vi "AddConstantPower.vi"(0 "deviceName":string, 1 "channel":u8, 2 "repeats":u16=1, 3 "power":sgl, 4 "samplingInterval":sgl, 5 "maxDuration":sgl, 6 "maxVoltage":sgl=inf, 7 "error in (no error)":errorcluster, 8 "isMaximumVoltageVsOCP":bool, 9 "minVoltage":sgl=-inf, 10 "isMinimumVoltageVsOCP":bool, 11 "maxCurrent":sgl=inf, 12 "minCurrent":sgl=-inf, 13 "maxCapacity":sgl=inf) -> (27 "error out":errorcluster)   [LabVIEW 2018]
doc: "EXPORT void AisAddConstantPower(const char* deviceName, uint8_t channel, uint16_t repeats, float power, float samplingInterval, float maxDuration, float maxVoltage, bool isMaximumVoltageVsOCP, float minVoltage, bool isMinimumVoltageVsOCP, float maxCurrent, float minCurrent, float maxCapacity);"
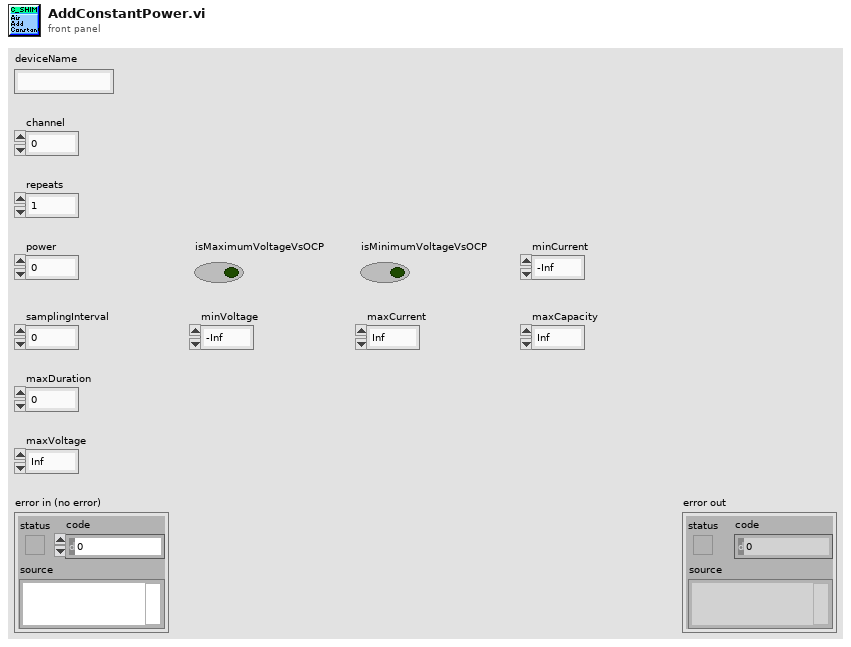
[diagram p1: front panel]
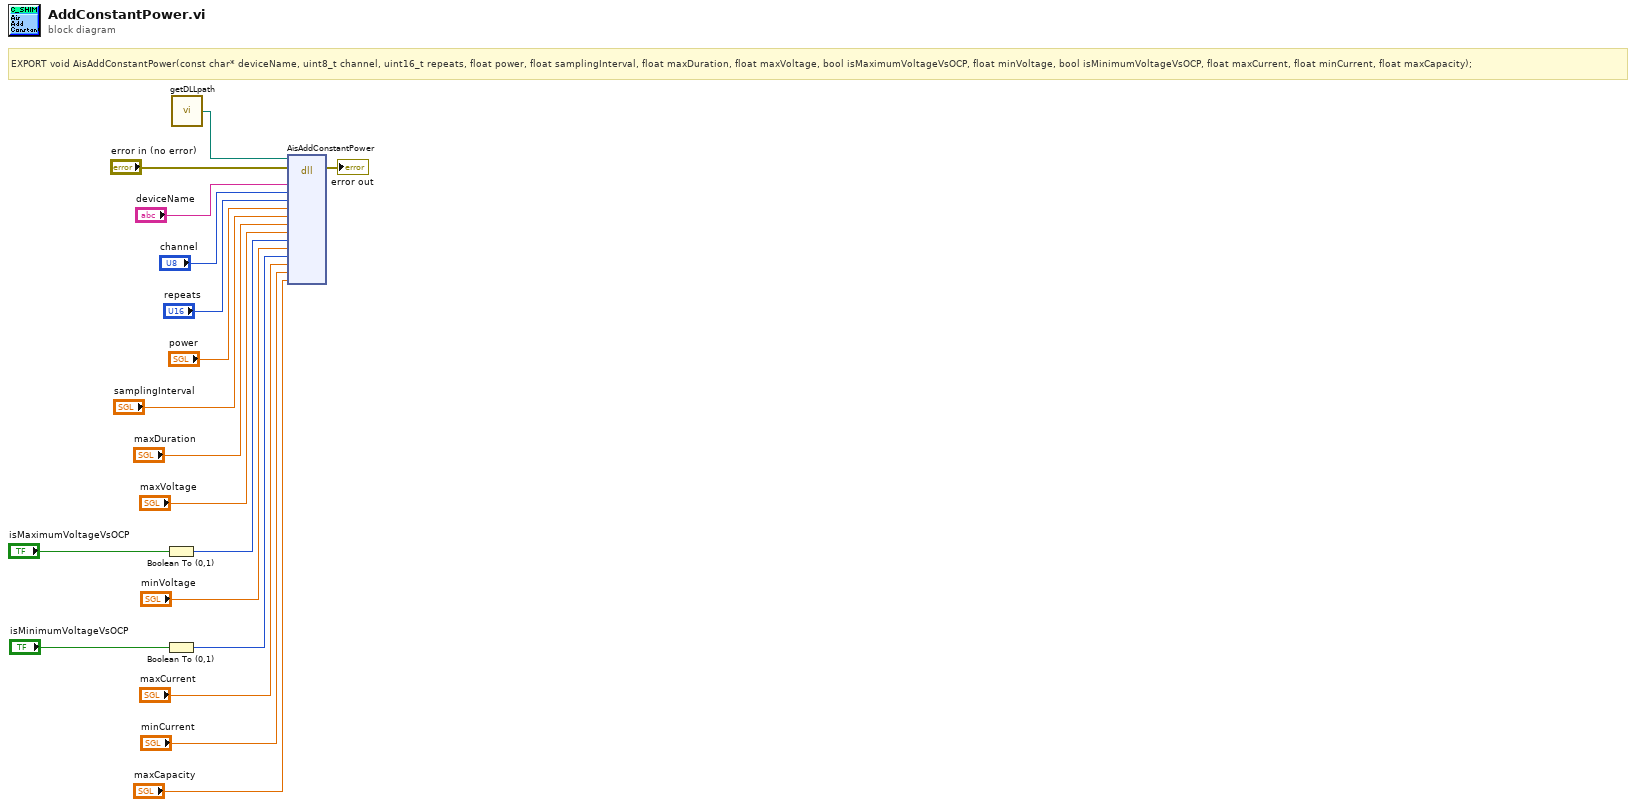
[diagram p0: block diagram]
diagram:
  # "EXPORT void AisAddConstantPower(const char* deviceName, uint8_t channel, uint16_t repeats, float power, float samplingInterval, float maxDuration, float maxVoltage, bool isMaximumVoltageVsOCP, float minVoltage, bool isMinimumVoltageVsOCP, float maxCurrent, float minCurrent, float maxCapacity);"
  n1 = Boolean To (0,1)(Boolean="isMaximumVoltageVsOCP") -> (0, 1=w10:i16)
  n2 = Boolean To (0,1)(Boolean="isMinimumVoltageVsOCP") -> (0, 1=w7:i16)
  n3 = call "getDLLpath.vi"() -> ("DLL_Path"=w1:path)
  n4 = dll-call lib="?" fn="AisAddConstantPower"(path in=w1, error in="error in (no error)", "deviceName"="deviceName", "channel"="channel", "repeats"="repeats", "power"="power", "samplingInterval"="samplingInterval", "maxDuration"="maxDuration", "maxVoltage"="maxVoltage", "isMaximumVoltageVsOCP"=w10, "minVoltage"="minVoltage", "isMinimumVoltageVsOCP"=w7, "maxCurrent"="maxCurrent", "minCurrent"="minCurrent", "maxCapacity"="maxCapacity") -> (error out=→"error out":errorcluster)  [unwired: 15 in, 1 out]
